vi "doACheck.vi"() -> ()   [LabVIEW 2014]
uses:
  <vilib>/Instr/_visa.llb/VISA Configure Serial Port (Instr).vi
  <vilib>/Instr/_visa.llb/VISA Flush IO Buffer Mask.ctl
  <vilib>/Utility/file.llb/Write To Spreadsheet File (DBL).vi
panel:
  out "error out":errorcluster
  out "Waveform Chart":dbl(graph)
  out "Distance, in":dbl
  out "return count":u32
  out "read buffer":string
  in  "VISA resource name":refnum<visa-resource-name>="COM3"
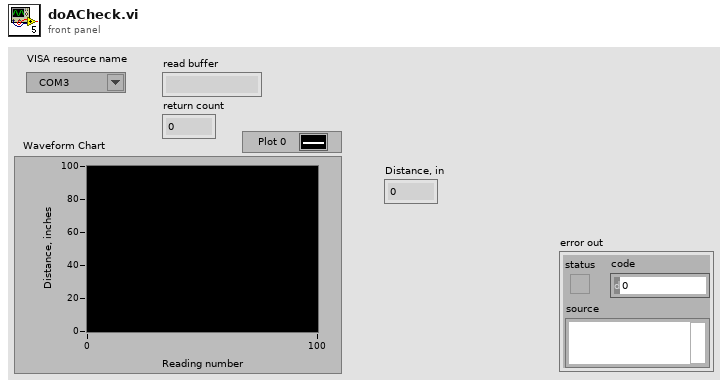
[diagram p1: front panel]
types:
  T1 = typedef "VISA Flush IO Buffer Mask.ctl" = u16
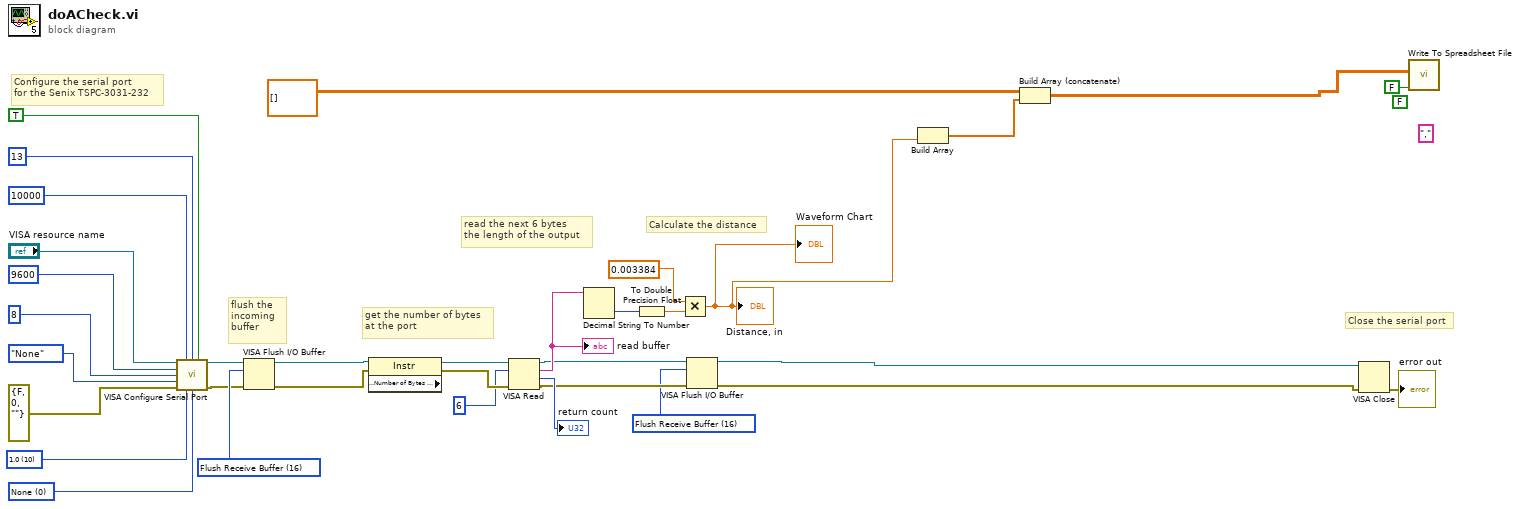
[diagram p0: block diagram]
diagram:
  (unwired) "," ("delimiter (\\t)")
  (unwired) FALSE ("transpose? (no:F)")
  w25 = T1 16 items=["Flush Receive Buffer"=16, "Write Transmit Buffer to Device"=32, "Flush Receive Buffer (No I/O)"=64, "Flush Transmit Buffer"=128] ("Mask")
  w11 = T1 16 items=["Flush Receive Buffer"=16, "Write Transmit Buffer to Device"=32, "Flush Receive Buffer (No I/O)"=64, "Flush Transmit Buffer"=128] ("Mask")
  w30 = u16 0 items=["None", "XON/XOFF", "RTS/CTS", "XON/XOFF & RTS/CTS", "DTR/DSR", "XON/XOFF & DTR/DSR"] ("flow control (0:none)")
  w32 = u16 10 items=["1.0"=10, "1.5"=15, "2.0"=20] ("stop bits (10: 1 bit)")
  # "Close the serial port"
  # "flush the \nincoming \nbuffer"
  # "Configure the serial port\nfor the Senix TSPC-3031-232"
  # "Calculate the distance"
  # "read the next 6 bytes\nthe length of the output"
  # "get the number of bytes\nat the port"
  n1 = call-poly "VISA Configure Serial Port"("VISA resource name"="VISA resource name", "timeout (10sec)"=u32 10000, "termination char\n(0xA = '\\n' = LF)"=u8 13 ("termination char\n(0xA = '\\n' = LF)"), "Enable Termination\nChar (T)"=TRUE ("Enable Termination\nChar (T)"), "baud rate (9600)"=u32 9600, "data bits (8)"=u16 8, "parity (0:none)"=enum16{"None", "Odd", "Even", "Mark", "Space"}."None", "error in (no error)"=errorcluster {"status"=FALSE, "code"=0, "source"=""}, "stop bits (10: 1 bit)"=w32, "flow control (0:none)"=w30) -> ("VISA resource name out"=w24:refnum<visa-resource-name>, "error out"=w23:errorcluster)  [unwired: 4 in]
  n2 = VISA Flush I/O Buffer(VISA resource name=w24, mask (16)=w25, error in (no error)=w23) -> (VISA resource name out=w4:refnum<visa-resource-name>, error out=w5:errorcluster)
  n3 = property class="Instr" props=["Serial Settings:Number of Bytes at Serial Port"](reference=w4, error in=w5) -> (reference out=w20:refnum<visa-resource-name>, error out=w19:errorcluster)  [unwired: 1 out]
  n4 = VISA Read(VISA resource name=w20, byte count=u32 6, error in (no error)=w19) -> (VISA resource name out=w13:refnum<visa-resource-name>, read buffer=w17:string, return count=→"return count":u32, error out=w12:errorcluster)
  "read buffer" <- w17
  n5 = Decimal String To Number(string=w17) -> (number=w16:i32)  [unwired: 2 in, 1 out]
  n6 = To Double Precision Float(number=w16) -> (double precision float=w15:dbl)
  n7 = Multiply(x=0.003384, y=w15) -> (x*y=w8:dbl)
  "Distance, in" <- w8
  "Waveform Chart" <- w8
  n8 = VISA Flush I/O Buffer(VISA resource name=w13, mask (16)=w11, error in (no error)=w12) -> (VISA resource name out=w2:refnum<visa-resource-name>, error out=w3:errorcluster)
  n9 = Build Array(w8) -> (w9:dbl[], w7:dbl)
  n10 = Build Array (concatenate)(dbl[][] [], w9) -> (w1:dbl[][])
  n11 = VISA Close(VISA resource name=w2, error in (no error)=w3) -> (error out=→"error out":errorcluster)
  n12 = call-poly <vilib>:"Write To Spreadsheet File.vi"("append to file? (new file:F)"=FALSE, "2D data"=w1) -> ("file path (dialog if empty)"=w21:path)  [unwired: 5 in, 1 out]
